vi "EOD Write(Older Version).vi"(9 "EODDataInput":T1(array[cluster]), 11 "Number of Waveforms":i32) -> (0 "error out":errorcluster, 2 "Iteration Test":i32, 3 "refnum out":refnum<file>)   [LabVIEW 2014]
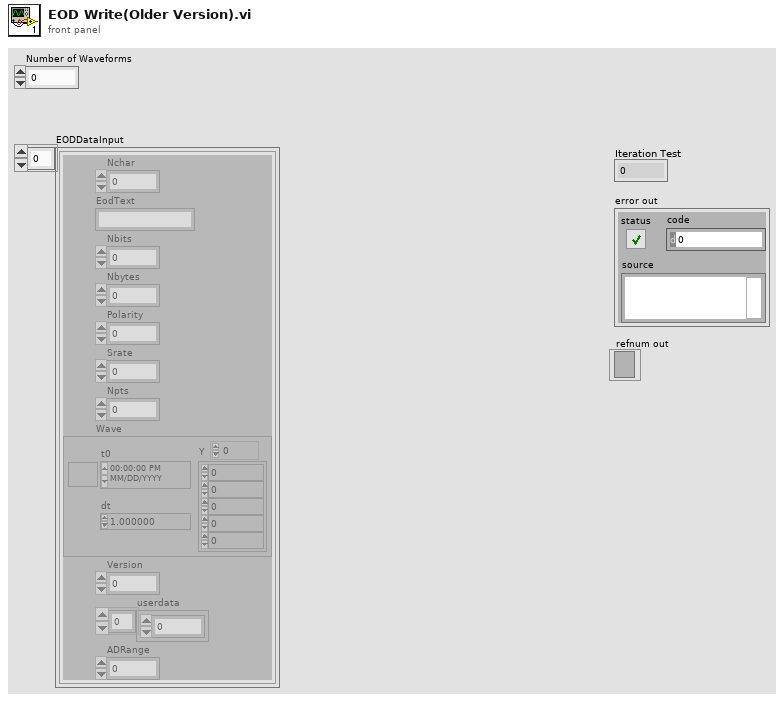
[diagram p1: front panel]
types:
  T1 = cluster{"Nchar":i32, "EodText":string, "Nbits":i32, "Nbytes":i32, "Polarity":i32, "Srate":i32, "Npts":i32, "Wave":waveform(dbl), "Version":i32, "userdata":dbl[], "ADRange":dbl}[]
  T2 = enum16{"open", "replace", "create", "open or create", "replace or create", "replace or create with confirmation"}
  T3 = enum16{"big-endian, network order", "native, host order", "little-endian"}
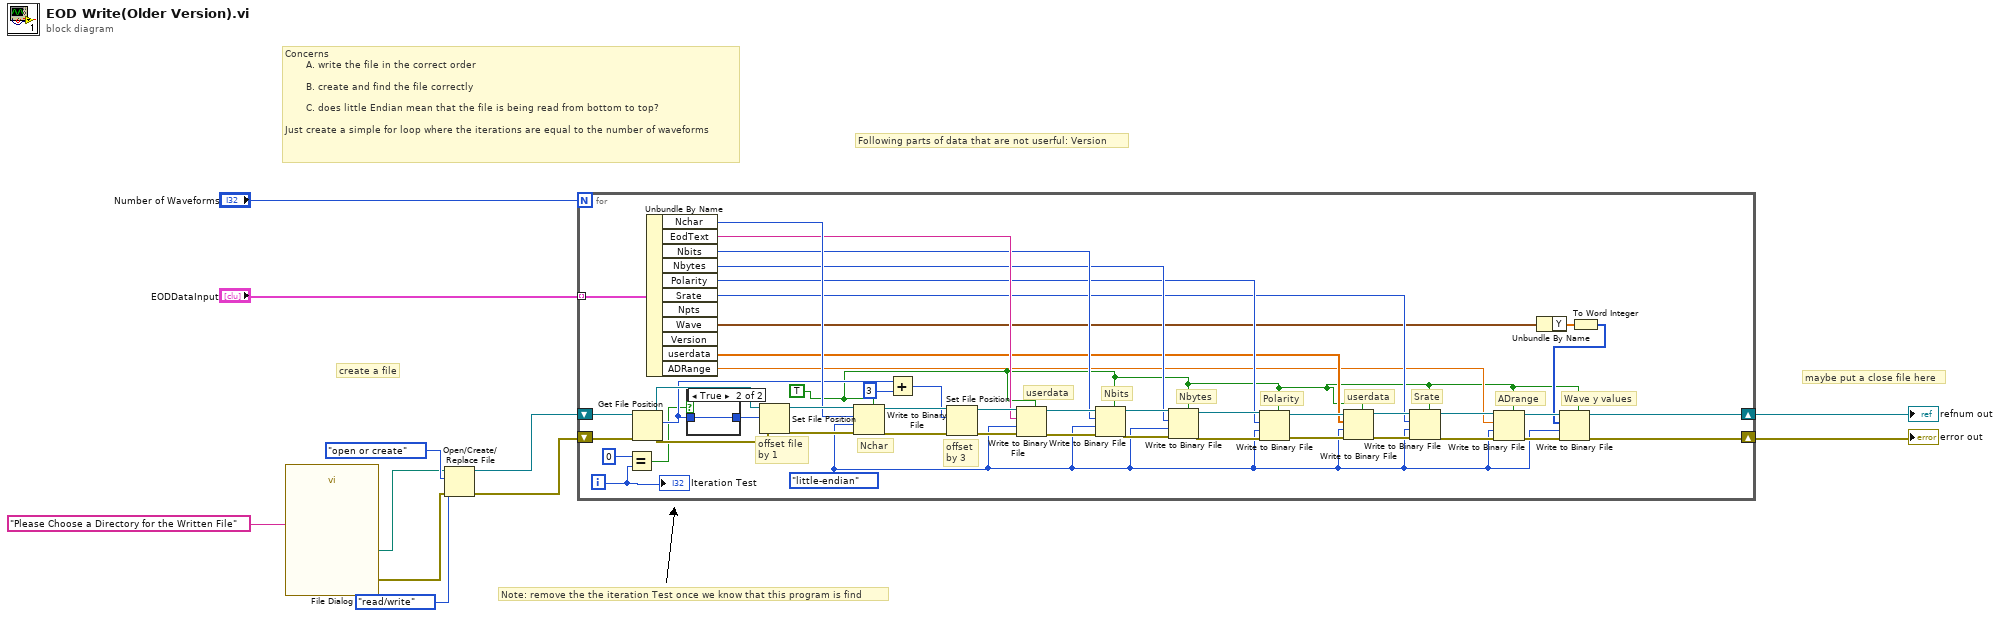
[diagram p0: block diagram]
diagram:
  # "maybe put a close file here"
  # "Note: remove the the iteration Test once we know that this program is find"
  # "Following parts of data that are not userful: Version"
  # "create a file"
  # "Concerns\n       A. write the file in the correct order\n\n       B. create and find the file correctly\n\n       C. does little Endian mean that the file is being read from bottom to top?\n\nJust create a simple for loop where the iterations are equal to the number of waveforms"
  n1 = call "File Dialog"("prompt"="Please Choose a Directory for the Written File") -> ("selected path"=w8:path, "error out"=w7:errorcluster)  [unwired: 11 in, 2 out]
  n2 = Open/Create/Replace File(file path (use dialog)=w8, error in=w7, operation (0:open)=T2."open or create", access (0:read/write)=enum16{"read/write", "read-only", "write-only"}."read/write") -> (refnum out=w5:refnum<file>, error out=w4:errorcluster)  [unwired: 2 in, 1 out]
  n3 = for {
    N: "Number of Waveforms" -> [_]
    tunnel: "EODDataInput" -> [w58] mode=indexing
    shift-right: [w22] -> w3
    shift-left: w5 -> [w21]
    shift-right: [w20] -> w2
    shift-left: w4 -> [w19]
    i -> [w15]
    w12 = TRUE
    w18 = T3."little-endian" ("byte order (0:big-endian, network order)")
    # "Wave y values"
    # "ADrange"
    # "Srate"
    # "userdata"
    # "Polarity"
    # "Nbytes"
    # "offset\nby 3"
    # "offset file\nby 1"
    # "Nchar"
    # "Nbits"
    # "userdata"
    n4 = Equal?(x=0, y=w15) -> (x = y?=w13:bool)
    n5 = Get File Position(4:w19, 7:w21) -> (0:w56:errorcluster, 2:w17:i64, 3:w57:refnum<file>)
    n6 = Unbundle By Name(w58) -> ("Nchar"=w53:i32, "EodText"=w46:string, "Nbits"=w43:i32, "Nbytes"=w38:i32, "Polarity"=w37:i32, "Srate"=w31:i32, "Wave"=w27:waveform(dbl), "userdata"=w34:dbl[], "ADRange"=w28:dbl)  [unwired: 2 out]
    n7 = case shown="True" w13 {
      tunnel: w17 -> [w59 w60]
      tunnel: [w59 w60] -> w16
      frame False {
      }
      frame True {
      }
    }
    n8 = Set File Position(offset (in bytes) (0)=w16, refnum=w57, error in=w56) -> (refnum out=w55:refnum<file>, error out=w54:errorcluster)  [unwired: 1 in]
    n9 = Write to Binary File(file (use dialog)=w55, data=w53, error in=w54, 5:w12, 9:w18) -> (refnum out=w52:refnum<file>, error out=w51:errorcluster)  [unwired: 1 in, 1 out]
    n10 = Add(x=w17, y=i64 3) -> (x+y=w50:i64)
    n11 = Set File Position(offset (in bytes) (0)=w50, refnum=w52, error in=w51) -> (refnum out=w48:refnum<file>, error out=w47:errorcluster)  [unwired: 1 in]
    n12 = Write to Binary File(file (use dialog)=w48, data=w46, error in=w47, 5:w12, 9:w18) -> (refnum out=w45:refnum<file>, error out=w44:errorcluster)  [unwired: 1 in, 1 out]
    n13 = Write to Binary File(file (use dialog)=w45, data=w43, error in=w44, 5:w12, 9:w18) -> (refnum out=w42:refnum<file>, error out=w41:errorcluster)  [unwired: 1 in, 1 out]
    n14 = Write to Binary File(file (use dialog)=w42, data=w38, error in=w41, 5:w12, 9:w18) -> (refnum out=w40:refnum<file>, error out=w39:errorcluster)  [unwired: 1 in, 1 out]
    n15 = Write to Binary File(file (use dialog)=w40, data=w37, error in=w39, 5:w12, 9:w18) -> (refnum out=w36:refnum<file>, error out=w35:errorcluster)  [unwired: 1 in, 1 out]
    n16 = Write to Binary File(file (use dialog)=w36, data=w34, error in=w35, 5:w12, 9:w18) -> (refnum out=w33:refnum<file>, error out=w32:errorcluster)  [unwired: 1 in, 1 out]
    n17 = Write to Binary File(file (use dialog)=w33, data=w31, error in=w32, 5:w12, 9:w18) -> (refnum out=w30:refnum<file>, error out=w29:errorcluster)  [unwired: 1 in, 1 out]
    n18 = Write to Binary File(file (use dialog)=w30, data=w28, error in=w29, 5:w12, 9:w18) -> (refnum out=w25:refnum<file>, error out=w24:errorcluster)  [unwired: 1 in, 1 out]
    n19 = Unbundle By Name(w27) -> ("Y"=w26:dbl[])
    n20 = To Word Integer(number=w26) -> (16bit integer=w23:i16[])
    n21 = Write to Binary File(file (use dialog)=w25, data=w23, error in=w24, 5:w12, 9:w18) -> (refnum out=w22:refnum<file>, error out=w20:errorcluster)  [unwired: 1 in, 1 out]
    "Iteration Test" <- w15
  }
  "refnum out" <- w3
  "error out" <- w2
